vi "OnOff Read.vi"(8 "error in":errorcluster, 11 "Cycler in":refnum<class "Cycler.lvclass">) -> (0 "error out":errorcluster, 1 "Changed or First Call?":bool, 2 "OnOff ACT":bool, 3 "Cycler out":refnum<class "Cycler.lvclass">)   [LabVIEW 2023, in "Cycler.lvclass"]
uses:
  Cycler.lvclass
  Cycler.lvclass/Cycler.ctl
  Low Level Capabilities/OnOff/OnOff.lvclass
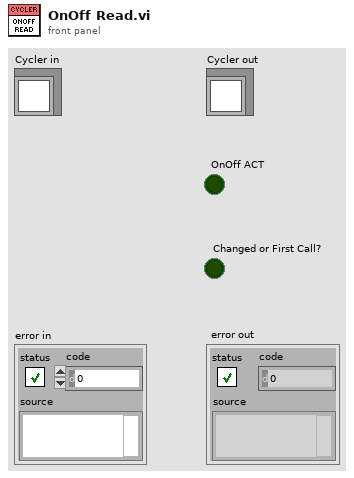
[diagram p1: front panel]
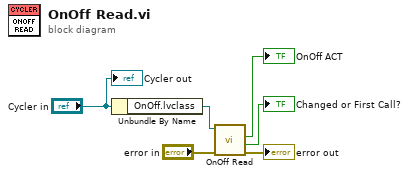
[diagram p0: block diagram]
diagram:
  n1 = Unbundle By Name("Cycler in") -> ("OnOff.lvclass"=w6:refnum<class "OnOff.lvclass">)
  n2 = call-dynamic "OnOff Read.vi"("error in"="error in", "OnOff in"=w6) -> ("error out"=→"error out":errorcluster, "Changed or First Call?"=→"Changed or First Call?":bool, "OnOff ACT"=→"OnOff ACT":bool)  [unwired: 6 in, 1 out]
  "Cycler out" <- "Cycler in"
